vi "GVSData View Global.vi"() -> ()   [LabVIEW 2013]
uses:
  Control/GVSGraph Event.ctl
  Control/GVSGraphView Property.ctl
  Control/GVSGraph Property.ctl
  Control/GVSDrag Graph.ctl
panel:
  in  "DragDrop Panel Idx":i32
  in  "DragDrop?":bool
  in  "DataViewPlotFinish":bool
  in  "Drag into Graph":T1
  in  "GraphView Property Array":T2[](array[typedef])
  in  "Graph Show Finish?":bool
  in  "Graph Queue Name":string
  in  "ChangeFlag":bool
  in  "Window Inserting...":bool
  in  "Active Graph VI Ref":refnum<vi>
  in  "Active Legend Ref":refnum<vi>
  in  "Plot Graph Loading":bool
  in  "Plot in Right Click?":bool
  in  "GraphEventCluster":T4
  in  "GraphDataType":u16(ring) items=["WAVE", "BAR1", "POLRA", "DIGITAL", "XY ", "BAR2", "EMPTY"]
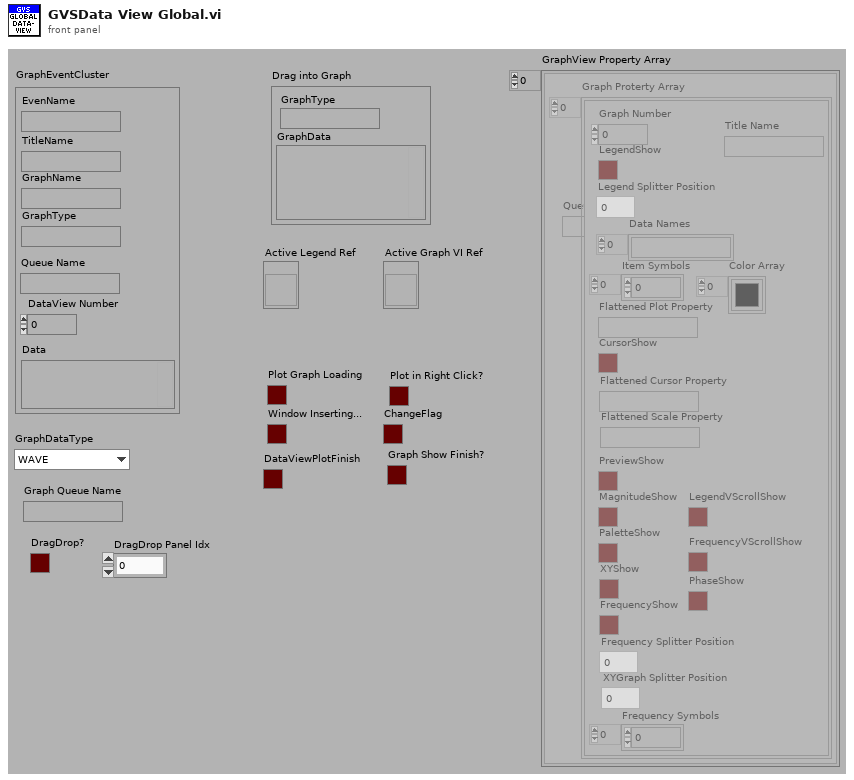
[diagram p1: front panel]
types:
  T1 = typedef "GVSDrag Graph.ctl" = cluster{"GraphType":string, "GraphData":variant}
  T2 = typedef "GVSGraphView Property.ctl" = cluster{"Queue Name":string, "Graph Proterty Array":T3[]}
  T3 = typedef "GVSGraph Property.ctl" = cluster{"LegendShow":bool, "Legend Splitter Position":dbl, "Data Names":string[], "Item Symbols":i32[], "Color Array":u32[], "Flattened Plot Property":string, "CursorShow":bool, "Flattened Cursor Property":string, "Graph Number":i32, "Flattened Scale Property":string, "PreviewShow":bool, "MagnitudeShow":bool, "PaletteShow":bool, "XYShow":bool, "FrequencyShow":bool, "Frequency Splitter Position":dbl, "XYGraph Splitter Position":dbl, "Frequency Symbols":i32[], "LegendVScrollShow":bool, "FrequencyVScrollShow":bool, "PhaseShow":bool, "Title Name":string}
  T4 = typedef "GVSGraph Event.ctl" = cluster{"EvenName":string, "TitleName":string, "GraphName":string, "GraphType":string, "Data":variant, "Queue Name":string, "DataView Number":i32}
diagram:
